vi "TCPClientInterfaceData.vi"(1 "信息":T2, 10 "客服接口枚举":enum16{"ini", "增", "删", "查", "改"}(ring)) -> (14 "客服表":T3(c390), 17 "查找结果":T1)   [LabVIEW 2019]
uses:
  02 Mode/TCPClientMode/TCPClientClass.lvclass
  <vilib>/Utility/miscctls.llb/LVMapReplaceAction.ctl
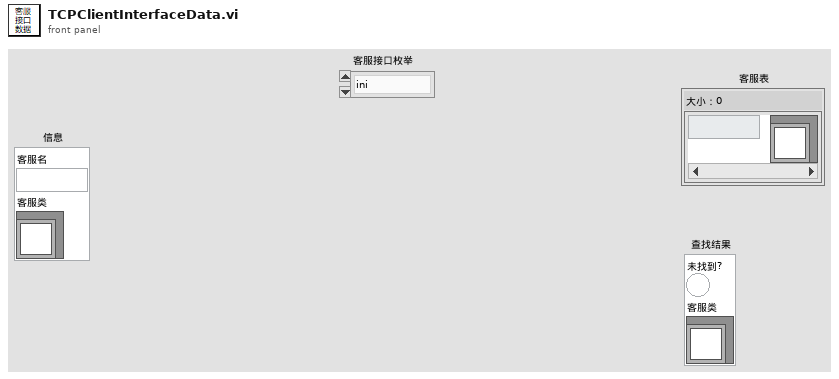
[diagram p1: front panel]
types:
  T1 = cluster{"未找到?":bool, "客服类":refnum<class "TCPClientClass.lvclass">}
  T2 = cluster{"客服名":string, "客服类":refnum<class "TCPClientClass.lvclass">}
  T3 = map{string, refnum<class "TCPClientClass.lvclass">}
  T4 = typedef "LVMapReplaceAction.ctl" = enum32{"Modify Entry only if found", "Add or Modify Entry", "Delete Entry"}
  T5 = cluster{"key not found?":bool, "TCPClientClass.lvclass":refnum<class "TCPClientClass.lvclass">}
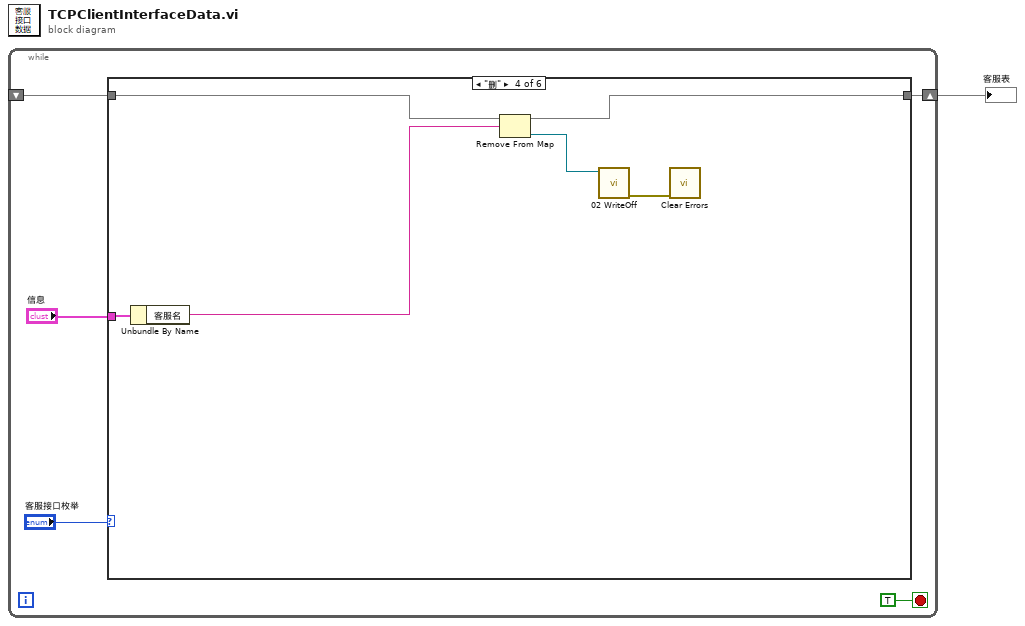
[diagram p0: block diagram]
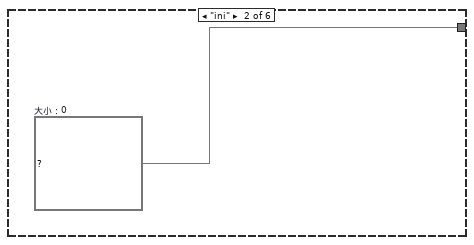
[diagram p3: hidden frame]
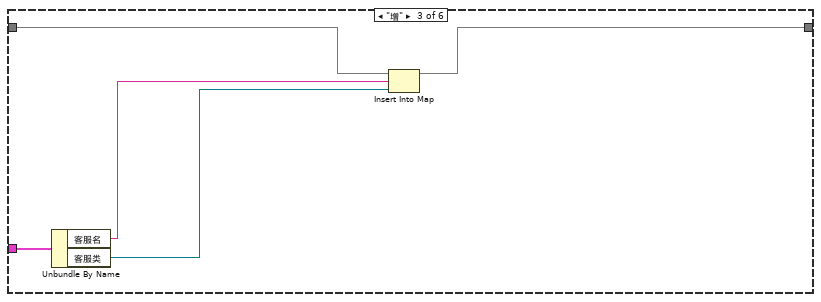
[diagram p4: hidden frame]
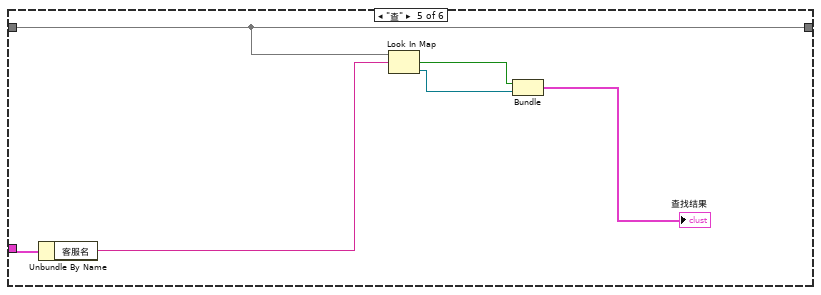
[diagram p5: hidden frame]
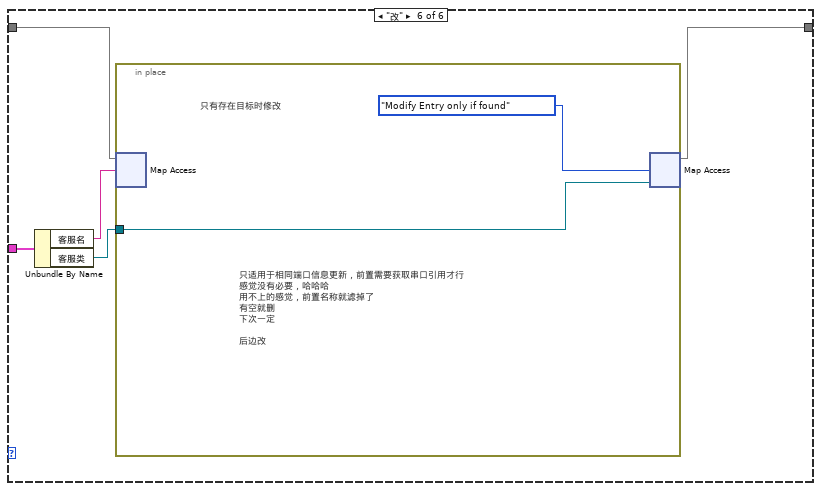
[diagram p6: hidden frame]
diagram:
  n1 = while {
    shift-right: [w4] -> w1
    shift-left: _ -> [w3]
    stop <- TRUE stop-if-true
    n2 = case shown="\"删\"" "客服接口枚举" {
      tunnel: [w7 w8 w12 w18 w23 w29] -> w4
      tunnel: w3 -> [w7 _ w13 w19 w23 w30]
      tunnel: "信息" -> [_ _ w11 w17 w25 w28]
      frame Default {
      }
      frame "ini" {
        w8 = T3 {}  # 大小：0
      }
      frame "增" {
        n3 = Unbundle By Name(w11) -> ("客服名"=w10:string, "客服类"=w9:refnum<class "TCPClientClass.lvclass">)
        n4 = Insert Into Map(map in=w13, key=w10, value=w9) -> (map out=w12:T3)  [unwired: 2 out]
      }
      frame "删" {
        n5 = Unbundle By Name(w17) -> ("客服名"=w16:string)
        n6 = Remove From Map(10:w16, 11:w19) -> (1:w15:refnum<class "TCPClientClass.lvclass">, 3:w18:T3)  [unwired: 1 out]
        n7 = call-dynamic "02 WriteOff.vi"("TCPClientClass 输入"=w15) -> ("error out"=w14:errorcluster)  [unwired: 9 in, 1 out]
        n8 = call <vilib>:"Clear Errors.vi"("error in (no error)"=w14) -> ()  [unwired: 5 in, 2 out]
      }
      frame "查" {
        n9 = Unbundle By Name(w25) -> ("客服名"=w24:string)
        n10 = Look In Map(map=w23, key=w24) -> (key not found?=w22:bool, value=w21:refnum<class "TCPClientClass.lvclass">)  [unwired: 1 in]
        n11 = Bundle("key not found?"=w22, "TCPClientClass.lvclass"=w21) -> (→"查找结果":T5)  [unwired: 1 in]
      }
      frame "改" {
        n12 = Unbundle By Name(w28) -> ("客服名"=w27:string, "客服类"=w26:refnum<class "TCPClientClass.lvclass">)
        n13 = in-place {
          in-place-border: w26 -> [w31]
          # "只适用于相同端口信息更新，前置需要获取串口引用才行\n感觉没有必要，哈哈哈\n用不上的感觉，前置名称就滤掉了\n有空就删\n下次一定\n\n后边改"
          # "只有存在目标时修改"
          n14 = in-place-map #1(w30, w27) -> ()  [unwired: 1 in, 2 out]
          n15 = in-place-map #1(w31, LVMapReplaceAction."Modify Entry only if found" ("操作")) -> (w29:T3)  [unwired: 2 out]
        }
      }
    }
  }
  "客服表" <- w1
